vi "MaxArrayDelayed.vi"(0 "Array":fxp<+/-,32,16>[](array[numeric]), 11 "Trigger":bool) -> (4 "Max":fxp<+/-,32,16> format="%.21g", 6 "Max Index":i32, 8 "Ready":bool, 10 "Min Index":i32, 15 "Min":fxp<+/-,32,16> format="%.21g")   [LabVIEW 2015]
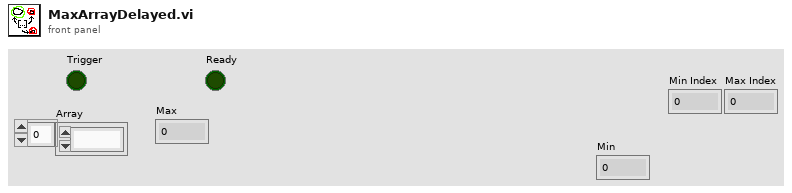
[diagram p1: front panel]
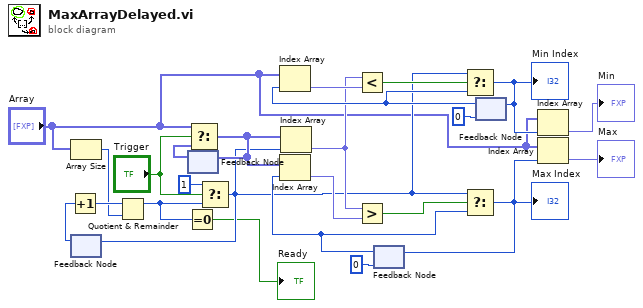
[diagram p0: block diagram]
diagram:
  n1 = Array Size(array="Array") -> (size(s)=w3:i32)
  n2 = feedback #1() -> (w21:i32)  [unwired: 1 in]
  n3 = Increment(x=w21) -> (x+1=w4:i32)
  n4 = Quotient & Remainder(x=w4, y=w3) -> (x-y*floor(x/y)=w2:i32)  [unwired: 1 out]
  n5 = Equal To 0?(x=w2) -> (x = 0?=→"Ready":bool)
  n6 = feedback #2() -> (w24:fxp<+/-,32,16>[])  [unwired: 1 in]
  n7 = Select(t="Array", s="Trigger", f=w24) -> (s? t:f=w13:fxp<+/-,32,16>[])
  n8 = feedback-in #2(w13) -> ()
  n9 = Select(t=u16 1, s="Trigger", f=w2) -> (s? t:f=w6:i32)
  n10 = feedback-in #1(w6) -> ()
  n11 = Index Array(array=w13, index=w6) -> (element=w9:fxp<+/-,32,16>)
  n12 = feedback #3(u16 0) -> (w14:i32)
  n13 = Index Array(array=w13, index=w14) -> (element=w12:fxp<+/-,32,16>)
  n14 = Greater?(x=w9, y=w12) -> (0:w7:bool)
  n15 = Select(t=w6, s=w7, f=w14) -> (s? t:f=w18:i32)
  "Max Index" <- w18
  n16 = feedback-in #3(w18) -> ()
  n17 = feedback #4(u16 0) -> (w11:i32)
  n18 = Index Array(array="Array", index=w11) -> (element=w10:fxp<+/-,32,16>)
  n19 = Less?(x=w9, y=w10) -> (x < y?=w8:bool)
  n20 = Select(t=w6, s=w8, f=w11) -> (s? t:f=w17:i32)
  "Min Index" <- w17
  n21 = feedback-in #4(w17) -> ()
  n22 = Index Array(array="Array", index=w17) -> (element=→"Min":fxp<+/-,32,16>)
  n23 = Index Array(array="Array", index=w18) -> (element=→"Max":fxp<+/-,32,16>)
